vi "FaulhaberV3-Ascii_V1.vi"() -> (1 "searchnames":string[](array[string]), 2 "ID":u32[](array[numeric]), 3 "Faulhaber Objects":T3(array[cluster]))   [LabVIEW 2011] (continued)
ype=\"7\" dataType=\"0005\" lowLimit=\"0\" highLimit=\"128\" accessType=\"rw\" defaultValue=\"0\" PDOmapping=\"RPDO\" objFlags=\"00020000\" />\n\t\t\t\t\t\t<CANopenSubObject subIndex=\"02\" name=\"Current feedforward delay\" objectType=\"7\" dataType=\"0006\" lowLimit=\"0\" highLimit=\"65535\" accessType=\"rw\" defaultValue=\"0\" PDOmapping=\"no\" objFlags=\"00020000\" />\n\t\t\t\t\t</CANopenObject>\n\t\t\t\t\t<CANopenObject index=\"234A\" name=\"Velocity feedforward parameters\" objectType=\"9\" subNumber=\"3\">\n\t\t\t\t\t\t<CANopenSubObject subIndex=\"00\" name=\"Number of entries\" objectType=\"7\" dataType=\"0005\" accessType=\"ro\" defaultValue=\"2\" PDOmapping=\"no\" />\n\t\t\t\t\t\t<CANopenSubObject subIndex=\"01\" name=\"Velocity feedforward factor\" objectType=\"7\" dataType=\"0005\" lowLimit=\"0\" highLimit=\"128\" accessType=\"rw\" defaultValue=\"0\" PDOmapping=\"RPDO\" objFlags=\"00020000\" />\n\t\t\t\t\t\t<CANopenSubObject subIndex=\"02\" name=\"Velocity feedforward delay\" objectType=\"7\" dataType=\"0006\" lowLimit=\"0\" highLimit=\"65535\" accessType=\"rw\" defaultValue=\"0\" PDOmapping=\"no\" objFlags=\"00020000\" />\n\t\t\t\t\t</CANopenObject>\n\t\t\t\t\t<CANopenObject index=\"234B\" name=\"Current filter parameters\" objectType=\"9\" subNumber=\"3\">\n\t\t\t\t\t\t<CANopenSubObject subIndex=\"00\" name=\"Number of entries\" objectType=\"7\" dataType=\"0005\" accessType=\"ro\" defaultValue=\"2\" PDOmapping=\"no\" />\n\t\t\t\t\t\t<CANopenSubObject subIndex=\"01\" name=\"Display current filter TF\" objectType=\"7\" dataType=\"0006\" lowLimit=\"0\" highLimit=\"65535\" accessType=\"rw\" PDOmapping=\"RPDO\" objFlags=\"00020000\" />\n\t\t\t\t\t\t<CANopenSubObject subIndex=\"02\" name=\"Display torque filter TF\" objectType=\"7\" dataType=\"0006\" lowLimit=\"0\" highLimit=\"65535\" accessType=\"rw\" PDOmapping=\"RPDO\" objFlags=\"00020000\" />\n\t\t\t\t\t</CANopenObject>\n\t\t\t\t\t<CANopenObject index=\"234C\" name=\"Current compensation parameters\" objectType=\"9\" subNumber=\"4\">\n\t\t\t\t\t\t<CANopenSubObject subIndex=\"00\" name=\"Number of entries\" objectType=\"7\" dataType=\"0005\" accessType=\"ro\" defaultValue=\"3\" PDOmapping=\"no\" />\n\t\t\t\t\t\t<CANopenSubObject subIndex=\"01\" name=\"Gravity compensation\" objectType=\"7\" dataType=\"0003\" lowLimit=\"-32768\" highLimit=\"32767\" accessType=\"rw\" defaultValue=\"0\" PDOmapping=\"RPDO\" objFlags=\"00020000\" />\n\t\t\t\t\t\t<CANopenSubObject subIndex=\"02\" name=\"Positive friction compensation\" objectType=\"7\" dataType=\"0006\" lowLimit=\"0\" highLimit=\"6000\" accessType=\"rw\" defaultValue=\"0\" PDOmapping=\"RPDO\" objFlags=\"00020000\" />\n\t\t\t\t\t\t<CANopenSubObject subIndex=\"03\" name=\"Negative friction compensation\" objectType=\"7\" dataType=\"0006\" lowLimit=\"0\" highLimit=\"6000\" accessType=\"rw\" defaultValue=\"0\" PDOmapping=\"RPDO\" objFlags=\"00020000\" />\n\t\t\t\t\t</CANopenObject>\n\t\t\t\t\t<CANopenObject index=\"2350\" name=\"Positive torque limit homing\" objectType=\"7\" dataType=\"0006\" lowLimit=\"0\" highLimit=\"6000\" accessType=\"rw\" defaultValue=\"1000\" PDOmapping=\"RPDO\" objFlags=\"00020000\" />\n\t\t\t\t\t<CANopenObject index=\"2351\" name=\"Negative torque limit homing\" objectType=\"7\" dataType=\"0006\" lowLimit=\"0\" highLimit=\"6000\" accessType=\"rw\" defaultValue=\"1000\" PDOmapping=\"RPDO\" objFlags=\"00020000\" />\n\t\t\t\t\t<CANopenObject index=\"2360\" name=\"Actual values\" objectType=\"9\" subNumber=\"11\">\n\t\t\t\t\t\t<CANopenSubObject subIndex=\"00\" name=\"Number of entries\" objectType=\"7\" dataType=\"0005\" accessType=\"ro\" defaultValue=\"10\" PDOmapping=\"no\" />\n\t\t\t\t\t\t<CANopenSubObject subIndex=\"01\" name=\"Motor current Id actual value\" objectType=\"7\" dataType=\"0003\" accessType=\"ro\" PDOmapping=\"TPDO\" />\n\t\t\t\t\t\t<CANopenSubObject subIndex=\"02\" name=\"Motor current Iq actual value\" objectType=\"7\" dataType=\"0003\" accessType=\"ro\" PDOmapping=\"TPDO\" />\n\t\t\t\t\t\t<CANopenSubObject subIndex=\"03\" name=\"Motor currrent IBlock actual value\" objectType=\"7\" dataType=\"0003\" accessType=\"ro\" PDOmapping=\"TPDO\" />\n\t\t\t\t\t\t<CANopenSubObject subIndex=\"04\" name=\"Motor current IDC actual value\" objectType=\"7\" dataType=\"0003\" accessType=\"ro\" PDOmapping=\"TPDO\" />\n\t\t\t\t\t\t<CANopenSubObject subIndex=\"05\" name=\"Velocity actual internal value\" objectType=\"7\" dataType=\"0003\" accessType=\"ro\" PDOmapping=\"TPDO\" />\n\t\t\t\t\t\t<CANopenSubObject subIndex=\"06\" name=\"Position actual internal value\" objectType=\"7\" dataType=\"0004\" accessType=\"ro\" PDOmapping=\"TPDO\" />\n\t\t\t\t\t\t<CANopenSubObject subIndex=\"07\" name=\"Actual commutation segment\" objectType=\"7\" dataType=\"0005\" accessType=\"ro\" PDOmapping=\"TPDO\" />\n\t\t\t\t\t\t<CANopenSubObject subIndex=\"08\" name=\"Actual commutation angle\" objectType=\"7\" dataType=\"0003\" accessType=\"ro\" PDOmapping=\"TPDO\" />\n\t\t\t\t\t\t<CANopenSubObject subIndex=\"09\" name=\"Reserved 9\" objectType=\"7\" dataType=\"0004\" accessType=\"ro\" PDOmapping=\"TPDO\" objFlags=\"00020003\" />\n\t\t\t\t\t\t<CANopenSubObject subIndex=\"0A\" name=\"Reserved 10\" objectType=\"7\" dataType=\"0004\" lowLimit=\"-2147483648\" highLimit=\"2147483647\" accessType=\"wo\" PDOmapping=\"no\" objFlags=\"00020003\" />\n\t\t\t\t\t</CANopenObject>\n\t\t\t\t\t<CANopenObject index=\"2370\" name=\"Trace configuration\" objectType=\"9\" subNumber=\"16\">\n\t\t\t\t\t\t<CANopenSubObject subIndex=\"00\" name=\"Number of entries\" objectType=\"7\" dataType=\"0005\" accessType=\"ro\" defaultValue=\"15\" PDOmapping=\"no\" />\n\t\t\t\t\t\t<CANopenSubObject subIndex=\"01\" name=\"Trigger value\" objectType=\"7\" dataType=\"0007\" lowLimit=\"0\" highLimit=\"4294967295\" accessType=\"rw\" defaultValue=\"0x00\" PDOmapping=\"no\" objFlags=\"00020000\" />\n\t\t\t\t\t\t<CANopenSubObject subIndex=\"02\" name=\"Trigger threshold\" objectType=\"7\" dataType=\"0004\" lowLimit=\"-2147483648\" highLimit=\"2147483647\" accessType=\"rw\" defaultValue=\"0\" PDOmapping=\"no\" objFlags=\"00020000\" />\n\t\t\t\t\t\t<CANopenSubObject subIndex=\"03\" name=\"Trigger offset\" objectType=\"7\" dataType=\"0003\" lowLimit=\"-32768\" highLimit=\"32767\" accessType=\"rw\" defaultValue=\"0\" PDOmapping=\"no\" objFlags=\"00020000\" />\n\t\t\t\t\t\t<CANopenSubObject subIndex=\"04\" name=\"Trigger mode\" objectType=\"7\" dataType=\"0006\" lowLimit=\"0\" highLimit=\"65535\" accessType=\"rw\" defaultValue=\"0\" PDOmapping=\"no\" objFlags=\"00020000\" />\n\t\t\t\t\t\t<CANopenSubObject subIndex=\"05\" name=\"Buffer length\" objectType=\"7\" dataType=\"0006\" lowLimit=\"1\" highLimit=\"2048\" accessType=\"rw\" defaultValue=\"2048\" PDOmapping=\"no\" objFlags=\"00020000\" />\n\t\t\t\t\t\t<CANopenSubObject subIndex=\"06\" name=\"Sample time\" objectType=\"7\" dataType=\"0005\" lowLimit=\"1\" highLimit=\"255\" accessType=\"rw\" defaultValue=\"1\" PDOmapping=\"no\" objFlags=\"00020000\" />\n\t\t\t\t\t\t<CANopenSubObject subIndex=\"07\" name=\"Trace source of channel 1\" objectType=\"7\" dataType=\"0007\" lowLimit=\"0\" highLimit=\"4294967295\" accessType=\"rw\" defaultValue=\"0x00\" PDOmapping=\"no\" objFlags=\"00020000\" />\n\t\t\t\t\t\t<CANopenSubObject subIndex=\"08\" name=\"Trace source of channel 2\" objectType=\"7\" dataType=\"0007\" lowLimit=\"0\" highLimit=\"4294967295\" accessType=\"rw\" defaultValue=\"0x00\" PDOmapping=\"no\" objFlags=\"00020000\" />\n\t\t\t\t\t\t<CANopenSubObject subIndex=\"09\" name=\"Trace source of channel 3\" objectType=\"7\" dataType=\"0007\" lowLimit=\"0\" highLimit=\"4294967295\" accessType=\"rw\" defaultValue=\"0x00\" PDOmapping=\"no\" objFlags=\"00020000\" />\n\t\t\t\t\t\t<CANopenSubObject subIndex=\"0A\" name=\"Trace source of channel 4\" objectType=\"7\" dataType=\"0007\" lowLimit=\"0\" highLimit=\"4294967295\" accessType=\"rw\" defaultValue=\"0x00\" PDOmapping=\"no\" objFlags=\"00020000\" />\n\t\t\t\t\t\t<CANopenSubObject subIndex=\"0B\" name=\"Monitor source of channel 1\" objectType=\"7\" dataType=\"0007\" lowLimit=\"0\" highLimit=\"4294967295\" accessType=\"rw\" defaultValue=\"0x00\" PDOmapping=\"no\" objFlags=\"00020000\" />\n\t\t\t\t\t\t<CANopenSubObject subIndex=\"0C\" name=\"Monitor source of channel 2\" objectType=\"7\" dataType=\"0007\" lowLimit=\"0\" highLimit=\"4294967295\" accessType=\"rw\" defaultValue=\"0x00\" PDOmapping=\"no\" objFlags=\"00020000\" />\n\t\t\t\t\t\t<CANopenSubObject subIndex=\"0D\" name=\"Monitor source of channel 3\" objectType=\"7\" dataType=\"0007\" lowLimit=\"0\" highLimit=\"4294967295\" accessType=\"rw\" defaultValue=\"0x00\" PDOmapping=\"no\" objFlags=\"00020000\" />\n\t\t\t\t\t\t<CANopenSubObject subIndex=\"0E\" name=\"Monitor source of channel 4\" objectType=\"7\" dataType=\"0007\" lowLimit=\"0\" highLimit=\"4294967295\" accessType=\"rw\" defaultValue=\"0x00\" PDOmapping=\"no\" objFlags=\"00020000\" />\n\t\t\t\t\t\t<CANopenSubObject subIndex=\"0F\" name=\"Extended recorder mode\" objectType=\"7\" dataType=\"0006\" lowLimit=\"0\" highLimit=\"65535\" accessType=\"wo\" defaultValue=\"0x00\" PDOmapping=\"no\" objFlags=\"00020000\" />\n\t\t\t\t\t</CANopenObject>\n\t\t\t\t\t<CANopenObject index=\"2371\" name=\"Trace buffer\" objectType=\"9\" subNumber=\"6\">\n\t\t\t\t\t\t<CANopenSubObject subIndex=\"00\" name=\"Number of entries\" objectType=\"7\" dataType=\"0005\" accessType=\"ro\" defaultValue=\"5\" PDOmapping=\"no\" />\n\t\t\t\t\t\t<CANopenSubObject subIndex=\"01\" name=\"Trace state\" objectType=\"7\" dataType=\"0006\" accessType=\"ro\" PDOmapping=\"no\" />\n\t\t\t\t\t\t<CANopenSubObject subIndex=\"02\" name=\"Trace value of channel 1\" objectType=\"2\" dataType=\"0009\" accessType=\"ro\" PDOmapping=\"no\" objFlags=\"0002\" />\n\t\t\t\t\t\t<CANopenSubObject subIndex=\"03\" name=\"Trace value of channel 2\" objectType=\"2\" dataType=\"0009\" accessType=\"ro\" PDOmapping=\"no\" objFlags=\"0002\" />\n\t\t\t\t\t\t<CANopenSubObject subIndex=\"04\" name=\"Trace value of channel 3\" objectType=\"2\" dataType=\"0009\" accessType=\"ro\" PDOmapping=\"no\" objFlags=\"0002\" />\n\t\t\t\t\t\t<CANopenSubObject subIndex=\"05\" name=\"Trace value of channel 4\" objectType=\"2\" dataType=\"0009\" accessType=\"ro\" PDOmapping=\"no\" objFlags=\"0002\" />\n\t\t\t\t\t</CANopenObject>\n\t\t\t\t\t<CANopenObject index=\"2372\" name=\"Logic trigger configuration\" objectType=\"9\" subNumber=\"3\">\n\t\t\t\t\t\t<CANopenSubObject subIndex=\"00\" name=\"Number of entries\" objectType=\"7\" dataType=\"0005\" accessType=\"ro\" defaultValue=\"2\" PDOmapping=\"no\" />\n\t\t\t\t\t\t<CANopenSubObject subIndex=\"01\" name=\"Logic trigger AND mask\" objectType=\"7\" dataType=\"0007\" lowLimit=\"0\" highLimit=\"4294967295\" accessType=\"rw\" defaultValue=\"0x00\" PDOmapping=\"no\" objFlags=\"00020000\" />\n\t\t\t\t\t\t<CANopenSubObject subIndex=\"02\" name=\"Logic trigger OR mask\" objectType=\"7\" dataType=\"0007\" lowLimit=\"0\" highLimit=\"4294967295\" accessType=\"rw\" defaultValue=\"0x00\" PDOmapping=\"no\" objFlags=\"00020000\" />\n\t\t\t\t\t</CANopenObject>\n\t\t\t\t\t<CANopenObject index=\"2373\" name=\"Event trigger configuration\" objectType=\"9\" subNumber=\"2\">\n\t\t\t\t\t\t<CANopenSubObject subIndex=\"00\" name=\"Number of entries\" objectType=\"7\" dataType=\"0005\" accessType=\"ro\" defaultValue=\"1\" PDOmapping=\"no\" />\n\t\t\t\t\t\t<CANopenSubObject subIndex=\"01\" name=\"Event trigger event selection\" objectType=\"7\" dataType=\"0006\" PDOmapping=\"no\" objFlags=\"00020000\" uniqueIDRef=\"UID_PARAM_237301\" />\n\t\t\t\t\t</CANopenObject>\n\t\t\t\t\t<CANopenObject index=\"2374\" name=\"Event flag configuration\" objectType=\"9\" subNumber=\"3\">\n\t\t\t\t\t\t<CANopenSubObject subIndex=\"00\" name=\"Number of entries\" objectType=\"7\" dataType=\"0005\" accessType=\"ro\" defaultValue=\"2\" PDOmapping=\"no\" />\n\t\t\t\t\t\t<CANopenSubObject subIndex=\"01\" name=\"Event flag set mask\" objectType=\"7\" dataType=\"0006\" lowLimit=\"0\" highLimit=\"65535\" accessType=\"rw\" defaultValue=\"0x0\" PDOmapping=\"no\" objFlags=\"00020000\" />\n\t\t\t\t\t\t<CANopenSubObject subIndex=\"02\" name=\"Event flag reset mask\" objectType=\"7\" dataType=\"0006\" lowLimit=\"0\" highLimit=\"65535\" accessType=\"rw\" defaultValue=\"0x0\" PDOmapping=\"no\" objFlags=\"00020000\" />\n\t\t\t\t\t</CANopenObject>\n\t\t\t\t\t<CANopenObject index=\"2378\" name=\"Trace channel configuration\" objectType=\"9\" subNumber=\"18\">\n\t\t\t\t\t\t<CANopenSubObject subIndex=\"00\" name=\"Number of entries\" objectType=\"7\" dataType=\"0005\" accessType=\"ro\" defaultValue=\"23\" PDOmapping=\"no\" />\n\t\t\t\t\t\t<CANopenSubObject subIndex=\"01\" name=\"Channel 1 filter time\" objectType=\"7\" dataType=\"0006\" lowLimit=\"0\" highLimit=\"65535\" accessType=\"rw\" defaultValue=\"0\" PDOmapping=\"RPDO\" objFlags=\"00020000\" />\n\t\t\t\t\t\t<CANopenSubObject subIndex=\"02\" name=\"Channel 1 sample time\" objectType=\"7\" dataType=\"0006\" lowLimit=\"0\" highLimit=\"65535\" accessType=\"rw\" defaultValue=\"1\" PDOmapping=\"RPDO\" objFlags=\"00020000\" />\n\t\t\t\t\t\t<CANopenSubObject subIndex=\"03\" name=\"Channel 1 number of samples\" objectType=\"7\" dataType=\"0006\" lowLimit=\"0\" highLimit=\"65535\" accessType=\"rw\" defaultValue=\"512\" PDOmapping=\"RPDO\" objFlags=\"00020000\" />\n\t\t\t\t\t\t<CANopenSubObject subIndex=\"04\" name=\"Channel 1 monitoring values\" objectType=\"7\" dataType=\"0006\" lowLimit=\"0\" highLimit=\"0x003F\" accessType=\"rw\" defaultValue=\"0\" PDOmapping=\"RPDO\" objFlags=\"00020000\" />\n\t\t\t\t\t\t<CANopenSubObject subIndex=\"05\" name=\"Channel 1 start event selection\" objectType=\"7\" dataType=\"0005\" PDOmapping=\"RPDO\" objFlags=\"00020000\" uniqueIDRef=\"UID_PARAM_237805\" />\n\t\t\t\t\t\t<CANopenSubObject subIndex=\"06\" name=\"Channel 1 update event selection\" objectType=\"7\" dataType=\"0005\" PDOmapping=\"RPDO\" objFlags=\"00020000\" uniqueIDRef=\"UID_PARAM_237806\" />\n\t\t\t\t\t\t<CANopenSubObject subIndex=\"07\" name=\"Channel 1 number of eval-cycles\" objectType=\"7\" dataType=\"0007\" lowLimit=\"0\" highLimit=\"4294967295\" accessType=\"rw\" defaultValue=\"0\" PDOmapping=\"TPDO\" objFlags=\"00020000\" />\n\t\t\t\t\t\t<CANopenSubObject subIndex=\"0E\" name=\"Channel 1 number of turnovers\" objectType=\"7\" dataType=\"0007\" accessType=\"ro\" PDOmapping=\"TPDO\" objFlags=\"00020000\" />\n\t\t\t\t\t\t<CANopenSubObject subIndex=\"0F\" name=\"Channel 1 done\" objectType=\"7\" dataType=\"0005\" accessType=\"ro\" PDOmapping=\"TPDO\" />\n\t\t\t\t\t\t<CANopenSubObject subIndex=\"10\" name=\"Channel 1 abs min value\" objectType=\"7\" dataType=\"0004\" accessType=\"ro\" defaultValue=\"2147483647\" PDOmapping=\"TPDO\" />\n\t\t\t\t\t\t<CANopenSubObject subIndex=\"11\" name=\"Channel 1 abs max value\" objectType=\"7\" dataType=\"0004\" accessType=\"ro\" defaultValue=\"-2147483648\" PDOmapping=\"TPDO\" />\n\t\t\t\t\t\t<CANopenSubObject subIndex=\"12\" name=\"Channel 1 minimum\" objectType=\"7\" dataType=\"0004\" accessType=\"ro\" PDOmapping=\"TPDO\" />\n\t\t\t\t\t\t<CANopenSubObject subIndex=\"13\" name=\"Channel 1 maximum\" objectType=\"7\" dataType=\"0004\" accessType=\"ro\" PDOmapping=\"TPDO\" />\n\t\t\t\t\t\t<CANopenSubObject subIndex=\"14\" name=\"Channel 1 mean value\" objectType=\"7\" dataType=\"0004\" accessType=\"ro\" PDOmapping=\"TPDO\" />\n\t\t\t\t\t\t<CANopenSubObject subIndex=\"15\" name=\"Channel 1 rms value\" objectType=\"7\" dataType=\"0004\" accessType=\"ro\" PDOmapping=\"TPDO\" />\n\t\t\t\t\t\t<CANopenSubObject subIndex=\"16\" name=\"Channel 1 period time\" objectType=\"7\" dataType=\"0007\" accessType=\"ro\" PDOmapping=\"TPDO\" />\n\t\t\t\t\t\t<CANopenSubObject subIndex=\"17\" name=\"Channel 1 sigma\" objectType=\"7\" dataType=\"0004\" accessType=\"ro\" PDOmapping=\"TPDO\" />\n\t\t\t\t\t</CANopenObject>\n\t\t\t\t\t<CANopenObject index=\"2379\" name=\"Trace channel configuration\" objectType=\"9\" subNumber=\"18\">\n\t\t\t\t\t\t<CANopenSubObject subIndex=\"00\" name=\"Number of entries\" objectType=\"7\" dataType=\"0005\" accessType=\"ro\" defaultValue=\"23\" PDOmapping=\"no\" />\n\t\t\t\t\t\t<CANopenSubObject subIndex=\"01\" name=\"Channel 2 filter time\" objectType=\"7\" dataType=\"0006\" lowLimit=\"0\" highLimit=\"65535\" accessType=\"rw\" defaultValue=\"0\" PDOmapping=\"RPDO\" objFlags=\"00020000\" />\n\t\t\t\t\t\t<CANopenSubObject subIndex=\"02\" name=\"Channel 2 sample time\" objectType=\"7\" dataType=\"0006\" lowLimit=\"0\" highLimit=\"65535\" accessType=\"rw\" defaultValue=\"1\" PDOmapping=\"RPDO\" objFlags=\"00020000\" />\n\t\t\t\t\t\t<CANopenSubObject subIndex=\"03\" name=\"Channel 2 number of samples\" objectType=\"7\" dataType=\"0006\" lowLimit=\"0\" highLimit=\"65535\" accessType=\"rw\" defaultValue=\"512\" PDOmapping=\"RPDO\" objFlags=\"00020000\" />\n\t\t\t\t\t\t<CANopenSubObject subIndex=\"04\" name=\"Channel 2 monitoring values\" objectType=\"7\" dataType=\"0006\" lowLimit=\"0\" highLimit=\"0x003F\" accessType=\"rw\" defaultValue=\"0\" PDOmapping=\"RPDO\" objFlags=\"00020000\" />\n\t\t\t\t\t\t<CANopenSubObject subIndex=\"05\" name=\"Channel 2 startevent selection\" objectType=\"7\" dataType=\"0005\" PDOmapping=\"RPDO\" objFlags=\"00020000\" uniqueIDRef=\"UID_PARAM_237905\" />\n\t\t\t\t\t\t<CANopenSubObject subIndex=\"06\" name=\"Channel 2 update event selection\" objectType=\"7\" dataType=\"0005\" PDOmapping=\"RPDO\" objFlags=\"00020000\" uniqueIDRef=\"UID_PARAM_237906\" />\n\t\t\t\t\t\t<CANopenSubObject subIndex=\"07\" name=\"Channel 2 number of eval-cycles\" objectType=\"7\" dataType=\"0007\" lowLimit=\"0\" highLimit=\"4294967295\" accessType=\"rw\" defaultValue=\"0\" PDOmapping=\"TPDO\" objFlags=\"00020000\" />\n\t\t\t\t\t\t<CANopenSubObject subIndex=\"0E\" name=\"Channel 2 number of turn-overs\" objectType=\"7\" dataType=\"0007\" accessType=\"ro\" PDOmapping=\"TPDO\" objFlags=\"00020000\" />\n\t\t\t\t\t\t<CANopenSubObject subIndex=\"0F\" name=\"Channel 2 done\" objectType=\"7\" dataType=\"0005\" accessType=\"ro\" PDOmapping=\"TPDO\" />\n\t\t\t\t\t\t<CANopenSubObject subIndex=\"10\" name=\"Channel 2 abs min value\" objectType=\"7\" dataType=\"0004\" accessType=\"ro\" defaultValue=\"2147483647\" PDOmapping=\"TPDO\" />\n\t\t\t\t\t\t<CANopenSubObject subIndex=\"11\" name=\"Channel 2 abs max value\" objectType=\"7\" dataType=\"0004\" accessType=\"ro\" defaultValue=\"-2147483648\" PDOmapping=\"TPDO\" />\n\t\t\t\t\t\t<CANopenSubObject subIndex=\"12\" name=\"Channel 2 minimum\" objectType=\"7\" dataType=\"0004\" accessType=\"ro\" PDOmapping=\"TPDO\" />\n\t\t\t\t\t\t<CANopenSubObject subIndex=\"13\" name=\"Channel 2 maximum\" objectType=\"7\" dataType=\"0004\" accessType=\"ro\" PDOmapping=\"TPDO\" />\n\t\t\t\t\t\t<CANopenSubObject subIndex=\"14\" name=\"Channel 2 mean value\" objectType=\"7\" dataType=\"0004\" accessType=\"ro\" PDOmapping=\"TPDO\" />\n\t\t\t\t\t\t<CANopenSubObject subIndex=\"15\" name=\"Channel 2 rms value\" objectType=\"7\" dataType=\"0004\" accessType=\"ro\" PDOmapping=\"TPDO\" />\n\t\t\t\t\t\t<CANopenSubObject subIndex=\"16\" name=\"Channel 2 period time\" objectType=\"7\" dataType=\"0007\" accessType=\"ro\" PDOmapping=\"TPDO\" />\n\t\t\t\t\t\t<CANopenSubObject subIndex=\"17\" name=\"Channel 2 sigma\" objectType=\"7\" dataType=\"0004\" accessType=\"ro\" PDOmapping=\"TPDO\" />\n\t\t\t\t\t</CANopenObject>\n\t\t\t\t\t<CANopenObject index=\"237A\" name=\"Trace channel configuration\" objectType=\"9\" subNumber=\"18\">\n\t\t\t\t\t\t<CANopenSubObject subIndex=\"00\" name=\"Number of entries\" objectType=\"7\" dataType=\"0005\" accessType=\"ro\" defaultValue=\"23\" PDOmapping=\"no\" />\n\t\t\t\t\t\t<CANopenSubObject subIndex=\"01\" name=\"Channel 3 filter time\" objectType=\"7\" dataType=\"0006\" lowLimit=\"0\" highLimit=\"65535\" accessType=\"rw\" defaultValue=\"0\" PDOmapping=\"RPDO\" objFlags=\"00020000\" />\n\t\t\t\t\t\t<CANopenSubObject subIndex=\"02\" name=\"Channel 3 sample time\" objectType=\"7\" dataType=\"0006\" lowLimit=\"0\" highLimit=\"65535\" accessType=\"rw\" defaultValue=\"1\" PDOmapping=\"RPDO\" objFlags=\"00020000\" />\n\t\t\t\t\t\t<CANopenSubObject subIndex=\"03\" name=\"Channel 3 number of samples\" objectType=\"7\" dataType=\"0006\" lowLimit=\"0\" highLimit=\"65535\" accessType=\"rw\" defaultValue=\"512\" PDOmapping=\"RPDO\" objFlags=\"00020000\" />\n\t\t\t\t\t\t<CANopenSubObject subIndex=\"04\" name=\"Channel 3 monitoring values\" objectType=\"7\" dataType=\"0006\" lowLimit=\"0\" highLimit=\"0x003F\" accessType=\"rw\" defaultValue=\"0\" PDOmapping=\"RPDO\" objFlags=\"00020000\" />\n\t\t\t\t\t\t<CANopenSubObject subIndex=\"05\" name=\"Channel 3 start event selection\" objectType=\"7\" dataType=\"0005\" PDOmapping=\"RPDO\" objFlags=\"00020000\" uniqueIDRef=\"UID_PARAM_237A05\" />\n\t\t\t\t\t\t<CANopenSubObject subIndex=\"06\" name=\"Channel 3 update event selection\" objectType=\"7\" dataType=\"0005\" PDOmapping=\"RPDO\" objFlags=\"00020000\" uniqueIDRef=\"UID_PARAM_237A06\" />\n\t\t\t\t\t\t<CANopenSubObject subIndex=\"07\" name=\"Channel 3 number of eval-cycles\" objectType=\"7\" dataType=\"0007\" lowLimit=\"0\" highLimit=\"4294967295\" accessType=\"rw\" defaultValue=\"0\" PDOmapping=\"TPDO\" objFlags=\"00020000\" />\n\t\t\t\t\t\t<CANopenSubObject subIndex=\"0E\" name=\"Channel 3 number of turn-overs\" objectType=\"7\" dataType=\"0007\" accessType=\"ro\" PDOmapping=\"TPDO\" objFlags=\"00020000\" />\n\t\t\t\t\t\t<CANopenSubObject subIndex=\"0F\" name=\"Channel 3 done\" objectType=\"7\" dataType=\"0005\" accessType=\"ro\" PDOmapping=\"TPDO\" />\n\t\t\t\t\t\t<CANopenSubObject subIndex=\"10\" name=\"Channel 3 abs min value\" objectType=\"7\" dataType=\"0004\" accessType=\"ro\" defaultValue=\"2147483647\" PDOmapping=\"TPDO\" />\n\t\t\t\t\t\t<CANopenSubObject subIndex=\"11\" name=\"Channel 3 abs max value\" objectType=\"7\" dataType=\"0004\" accessType=\"ro\" defaultValue=\"-2147483648\" PDOmapping=\"TPDO\" />\n\t\t\t\t\t\t<CANopenSubObject subIndex=\"12\" name=\"Channel 3 minimum\" objectType=\"7\" dataType=\"0004\" accessType=\"ro\" PDOmapping=\"TPDO\" />\n\t\t\t\t\t\t<CANopenSubObject subIndex=\"13\" name=\"Channel 3 maximum\" objectType=\"7\" dataType=\"0004\" accessType=\"ro\" PDOmapping=\"TPDO\" />\n\t\t\t\t\t\t<CANopenSubObject subIndex=\"14\" name=\"Channel 3 mean value\" objectType=\"7\" dataType=\"0004\" accessType=\"ro\" PDOmapping=\"TPDO\" />\n\t\t\t\t\t\t<CANopenSubObject subIndex=\"15\" name=\"Channel 3 rms value\" objectType=\"7\" dataType=\"0004\" accessType=\"ro\" PDOmapping=\"TPDO\" />\n\t\t\t\t\t\t<CANopenSubObject subIndex=\"16\" name=\"Channel 3 period time\" objectType=\"7\" dataType=\"0007\" accessType=\"ro\" PDOmapping=\"TPDO\" />\n\t\t\t\t\t\t<CANopenSubObject subIndex=\"17\" name=\"Channel 3 sigma\" objectType=\"7\" dataType=\"0004\" accessType=\"ro\" PDOmapping=\"TPDO\" />\n\t\t\t\t\t</CANopenObject>\n\t\t\t\t\t<CANopenObject index=\"237B\" name=\"Trace channel configuration\" objectType=\"9\" subNumber=\"18\">\n\t\t\t\t\t\t<CANopenSubObject subIndex=\"00\" name=\"Number of entries\" objectType=\"7\" dataType=\"0005\" accessType=\"ro\" defaultValue=\"23\" PDOmapping=\"no\" />\n\t\t\t\t\t\t<CANopenSubObject subIndex=\"01\" name=\"Channel 4 filter time\" objectType=\"7\" dataType=\"0006\" lowLimit=\"0\" highLimit=\"65535\" accessType=\"rw\" defaultValue=\"0\" PDOmapping=\"RPDO\" objFlags=\"00020000\" />\n\t\t\t\t\t\t<CANopenSubObject subIndex=\"02\" name=\"Channel 4 sample time\" objectType=\"7\" dataType=\"0006\" lowLimit=\"0\" highLimit=\"65535\" accessType=\"rw\" defaultValue=\"1\" PDOmapping=\"RPDO\" objFlags=\"00020000\" />\n\t\t\t\t\t\t<CANopenSubObject subIndex=\"03\" name=\"Channel 4 number of samples\" objectType=\"7\" dataType=\"0006\" lowLimit=\"0\" highLimit=\"65535\" accessType=\"rw\" defaultValue=\"512\" PDOmapping=\"RPDO\" objFlags=\"00020000\" />\n\t\t\t\t\t\t<CANopenSubObject subIndex=\"04\" name=\"Channel 4 monitoring values\" objectType=\"7\" dataType=\"0006\" lowLimit=\"0\" highLimit=\"0x003F\" accessType=\"rw\" defaultValue=\"0\" PDOmapping=\"RPDO\" objFlags=\"00020000\" />\n\t\t\t\t\t\t<CANopenSubObject subIndex=\"05\" name=\"Channel 4 start event selection\" objectType=\"7\" dataType=\"0005\" PDOmapping=\"RPDO\" objFlags=\"00020000\" uniqueIDRef=\"UID_PARAM_237B05\" />\n\t\t\t\t\t\t<CANopenSubObject subIndex=\"06\" name=\"Channel 4 update event selection\" objectType=\"7\" dataType=\"0005\" PDOmapping=\"RPDO\" objFlags=\"00020000\" uniqueIDRef=\"UID_PARAM_237B06\" />\n\t\t\t\t\t\t<CANopenSubObject subIndex=\"07\" name=\"Channel 4 number of eval-cycles\" objectType=\"7\" dataType=\"0007\" lowLimit=\"0\" highLimit=\"4294967295\" accessType=\"rw\" defaultValue=\"0\" PDOmapping=\"TPDO\" objFlags=\"00020000\" />\n\t\t\t\t\t\t<CANopenSubObject subIndex=\"0E\" name=\"Channel 4 number of turn-overs\" objectType=\"7\" dataType=\"0007\" accessType=\"ro\" PDOmapping=\"TPDO\" objFlags=\"00020000\" />\n\t\t\t\t\t\t<CANopenSubObject subIndex=\"0F\" name=\"Channel 4 done\" objectType=\"7\" dataType=\"0005\" accessType=\"ro\" PDOmapping=\"TPDO\" />\n\t\t\t\t\t\t<CANopenSubObject subIndex=\"10\" name=\"Channel 4 abs min value\" objectType=\"7\" dataType=\"0004\" accessType=\"ro\" defaultValue=\"2147483647\" PDOmapping=\"TPDO\" />\n\t\t\t\t\t\t<CANopenSubObject subIndex=\"11\" name=\"Channel 4 abs max value\" objectType=\"7\" dataType=\"0004\" accessType=\"ro\" defaultValue=\"-2147483648\" PDOmapping=\"TPDO\" />\n\t\t\t\t\t\t<CANopenSubObject subIndex=\"12\" name=\"Channel 4 minimum\" objectType=\"7\" dataType=\"0004\" accessType=\"ro\" PDOmapping=\"TPDO\" />\n\t\t\t\t\t\t<CANopenSubObject subIndex=\"13\" name=\"Channel 4 maximum\" objectType=\"7\" dataType=\"0004\" accessType=\"ro\" PDOmapping=\"TPDO\" />\n\t\t\t\t\t\t<CANopenSubObject subIndex=\"14\" name=\"Channel 4 mean value\" objectType=\"7\" dataType=\"0004\" accessType=\"ro\" PDOmapping=\"TPDO\" />\n\t\t\t\t\t\t<CANopenSubObject subIndex=\"15\" name=\"Channel 4 rms value\" objectType=\"7\" dataType=\"0004\" accessType=\"ro\" PDOmapping=\"TPDO\" />\n\t\t\t\t\t\t<CANopenSubObject subIndex=\"16\" name=\"Channel 4 period time\" objectType=\"7\" dataType=\"0007\" accessType=\"ro\" PDOmapping=\"TPDO\" />\n\t\t\t\t\t\t<CANopenSubObject subIndex=\"17\" name=\"Channel 4 sigma\" objectType=\"7\" dataType=\"0004\" accessType=\"ro\" PDOmapping=\"TPDO\" />\n\t\t\t\t\t</CANopenObject>\n\t\t\t\t\t<CANopenObject index=\"2380\" name=\"PRBS generator\" objectType=\"9\" subNumber=\"6\">\n\t\t\t\t\t\t<CANopenSubObject subIndex=\"00\" name=\"Number of entries\" objectType=\"7\" dataType=\"0005\" accessType=\"ro\" defaultValue=\"5\" PDOmapping=\"no\" objFlags=\"00020002\" />\n\t\t\t\t\t\t<CANopenSubObject subIndex=\"01\" name=\"Shift register init\" objectType=\"7\" dataType=\"0006\" lowLimit=\"0\" highLimit=\"65535\" accessType=\"rw\" PDOmapping=\"no\" objFlags=\"00020002\" />\n\t\t\t\t\t\t<CANopenSubObject subIndex=\"02\" name=\"Gain\" objectType=\"7\" dataType=\"0003\" lowLimit=\"-32768\" highLimit=\"32767\" accessType=\"rw\" PDOmapping=\"no\" objFlags=\"00020002\" />\n\t\t\t\t\t\t<CANopenSubObject subIndex=\"03\" name=\"Offset\" objectType=\"7\" dataType=\"0003\" lowLimit=\"-32768\" highLimit=\"32767\" accessType=\"rw\" PDOmapping=\"no\" objFlags=\"00020002\" />\n\t\t\t\t\t\t<CANopenSubObject subIndex=\"04\" name=\"Sample rate factor\" objectType=\"7\" dataType=\"0005\" lowLimit=\"0\" highLimit=\"255\" accessType=\"rw\" PDOmapping=\"no\" objFlags=\"00020002\" />\n\t\t\t\t\t\t<CANopenSubObject subIndex=\"05\" name=\"Enable\" objectType=\"7\" dataType=\"0005\" lowLimit=\"0\" highLimit=\"255\" accessType=\"rw\" PDOmapping=\"no\" objFlags=\"00020002\" />\n\t\t\t\t\t</CANopenObject>\n\t\t\t\t\t<CANopenObject index=\"2381\" name=\"Start up generator\" objectType=\"9\" subNumber=\"9\">\n\t\t\t\t\t\t<CANopenSubObject subIndex=\"00\" name=\"Number of entries\" objectType=\"7\" dataType=\"0005\" accessType=\"ro\" defaultValue=\"8\" PDOmapping=\"no\" objFlags=\"00020002\" />\n\t\t\t\t\t\t<CANopenSubObject subIndex=\"01\" name=\"Speed threshold\" objectType=\"7\" dataType=\"0006\" lowLimit=\"0\" highLimit=\"65535\" accessType=\"rw\" PDOmapping=\"no\" objFlags=\"00020002\" />\n\t\t\t\t\t\t<CANopenSubObject subIndex=\"02\" name=\"Timeout time\" objectType=\"7\" dataType=\"0007\" lowLimit=\"0\" highLimit=\"4294967295\" accessType=\"rw\" PDOmapping=\"no\" objFlags=\"00020002\" />\n\t\t\t\t\t\t<CANopenSubObject subIndex=\"03\" name=\"Target value\" objectType=\"7\" dataType=\"0006\" lowLimit=\"0\" highLimit=\"65535\" accessType=\"rw\" PDOmapping=\"no\" objFlags=\"00020002\" />\n\t\t\t\t\t\t<CANopenSubObject subIndex=\"04\" name=\"Reset\" objectType=\"7\" dataType=\"0005\" lowLimit=\"0\" highLimit=\"255\" accessType=\"rw\" PDOmapping=\"no\" objFlags=\"00020002\" />\n\t\t\t\t\t\t<CANopenSubObject subIndex=\"05\" name=\"Enable\" objectType=\"7\" dataType=\"0005\" lowLimit=\"0\" highLimit=\"255\" accessType=\"rw\" PDOmapping=\"no\" objFlags=\"00020002\" />\n\t\t\t\t\t\t<CANopenSubObject subIndex=\"06\" name=\"Ready\" objectType=\"7\" dataType=\"0007\" lowLimit=\"0\" highLimit=\"4294967295\" accessType=\"rw\" PDOmapping=\"no\" objFlags=\"00020002\" />\n\t\t\t\t\t\t<CANopenSubObject subIndex=\"07\" name=\"TimeThreshold\" objectType=\"7\" dataType=\"0007\" lowLimit=\"0\" highLimit=\"4294967295\" accessType=\"rw\" PDOmapping=\"no\" objFlags=\"00020002\" />\n\t\t\t\t\t\t<CANopenSubObject subIndex=\"08\" name=\"Iteration\" objectType=\"7\" dataType=\"0007\" lowLimit=\"0\" highLimit=\"4294967295\" accessType=\"rw\" PDOmapping=\"no\" objFlags=\"00020002\" />\n\t\t\t\t\t</CANopenObject>\n\t\t\t\t\t<CANopenObject index=\"2382\" name=\"Sinusoidal excitation\" objectType=\"9\" subNumber=\"4\">\n\t\t\t\t\t\t<CANopenSubObject subIndex=\"00\" name=\"Number of entries\" objectType=\"7\" dataType=\"0005\" accessType=\"ro\" defaultValue=\"3\" PDOmapping=\"no\" objFlags=\"00020002\" />\n\t\t\t\t\t\t<CANopenSubObject subIndex=\"01\" name=\"Amplitude\" objectType=\"7\" dataType=\"0006\" lowLimit=\"0\" highLimit=\"65535\" accessType=\"rw\" PDOmapping=\"no\" objFlags=\"00020002\" />\n\t\t\t\t\t\t<CANopenSubObject subIndex=\"02\" name=\"Frequency\" objectType=\"7\" dataType=\"0006\" lowLimit=\"0\" highLimit=\"65535\" accessType=\"rw\" PDOmapping=\"no\" objFlags=\"00020002\" />\n\t\t\t\t\t\t<CANopenSubObject subIndex=\"03\" name=\"Enable\" objectType=\"7\" dataType=\"0005\" lowLimit=\"0\" highLimit=\"255\" accessType=\"rw\" PDOmapping=\"no\" objFlags=\"00020002\" />\n\t\t\t\t\t</CANopenObject>\n\t\t\t\t\t<CANopenObject index=\"238F\" name=\"Select signal generator source\" objectType=\"9\" subNumber=\"2\">\n\t\t\t\t\t\t<CANopenSubObject subIndex=\"00\" name=\"Number of entries\" objectType=\"7\" dataType=\"0005\" accessType=\"ro\" defaultValue=\"1\" PDOmapping=\"no\" objFlags=\"00020002\" />\n\t\t\t\t\t\t<CANopenSubObject subIndex=\"01\" name=\"Selector\" objectType=\"7\" dataType=\"0005\" lowLimit=\"0\" highLimit=\"255\" accessType=\"rw\" defaultValue=\"0\" PDOmapping=\"no\" objFlags=\"00020002\" />\n\t\t\t\t\t</CANopenObject>\n\t\t\t\t\t<CANopenObject index=\"23F0\" name=\"23F0_00\" objectType=\"9\" subNumber=\"7\">\n\t\t\t\t\t\t<CANopenSubObject subIndex=\"00\" name=\"Number of entries\" objectType=\"7\" dataType=\"0005\" accessType=\"ro\" defaultValue=\"6\" PDOmapping=\"no\" objFlags=\"00020003\" />\n\t\t\t\t\t\t<CANopenSubObject subIndex=\"01\" name=\"23F0_01\" objectType=\"7\" dataType=\"0007\" accessType=\"ro\" PDOmapping=\"no\" objFlags=\"00020003\" />\n\t\t\t\t\t\t<CANopenSubObject subIndex=\"02\" name=\"23F0_02\" objectType=\"7\" dataType=\"0005\" accessType=\"ro\" PDOmapping=\"no\" objFlags=\"00020003\" />\n\t\t\t\t\t\t<CANopenSubObject subIndex=\"03\" name=\"23F0_03\" objectType=\"7\" dataType=\"0005\" accessType=\"ro\" PDOmapping=\"no\" objFlags=\"00020003\" />\n\t\t\t\t\t\t<CANopenSubObject subIndex=\"04\" name=\"23F0_04\" objectType=\"7\" dataType=\"0006\" accessType=\"ro\" PDOmapping=\"no\" objFlags=\"00020003\" />\n\t\t\t\t\t\t<CANopenSubObject subIndex=\"05\" name=\"23F0_05\" objectType=\"7\" dataType=\"0007\" accessType=\"ro\" PDOmapping=\"no\" objFlags=\"00020003\" />\n\t\t\t\t\t\t<CANopenSubObject subIndex=\"06\" name=\"23F0_06\" objectType=\"7\" dataType=\"0007\" accessType=\"ro\" PDOmapping=\"no\" objFlags=\"00020003\" />\n\t\t\t\t\t</CANopenObject>\n\t\t\t\t\t<CANopenObject index=\"23F1\" name=\"23F1_00\" objectType=\"9\" subNumber=\"3\">\n\t\t\t\t\t\t<CANopenSubObject subIndex=\"00\" name=\"Number of entries\" objectType=\"7\" dataType=\"0005\" accessType=\"ro\" defaultValue=\"2\" PDOmapping=\"no\" objFlags=\"00020003\" />\n\t\t\t\t\t\t<CANopenSubObject subIndex=\"01\" name=\"23F1_01\" objectType=\"7\" dataType=\"0004\" accessType=\"ro\" PDOmapping=\"no\" objFlags=\"00020003\" />\n\t\t\t\t\t\t<CANopenSubObject subIndex=\"02\" name=\"23F1_02\" objectType=\"7\" dataType=\"0004\" accessType=\"ro\" PDOmapping=\"no\" objFlags=\"00020003\" />\n\t\t\t\t\t</CANopenObject>\n\t\t\t\t\t<CANopenObject index=\"23F3\" name=\"23F2_00 \" objectType=\"9\" subNumber=\"6\">\n\t\t\t\t\t\t<CANopenSubObject subIndex=\"00\" name=\"Number of entries\" objectType=\"7\" dataType=\"0005\" accessType=\"ro\" defaultValue=\"5\" PDOmapping=\"no\" objFlags=\"0003\" />\n\t\t\t\t\t\t<CANopenSubObject subIndex=\"01\" name=\"Actual state\" objectType=\"7\" dataType=\"0002\" accessType=\"ro\" PDOmapping=\"no\" objFlags=\"0003\" />\n\t\t\t\t\t\t<CANopenSubObject subIndex=\"02\" name=\"Demand position\" objectType=\"7\" dataType=\"0004\" accessType=\"ro\" PDOmapping=\"no\" objFlags=\"0003\" />\n\t\t\t\t\t\t<CANopenSubObject subIndex=\"03\" name=\"Demand speed\" objectType=\"7\" dataType=\"0004\" accessType=\"ro\" PDOmapping=\"no\" objFlags=\"0003\" />\n\t\t\t\t\t\t<CANopenSubObject subIndex=\"04\" name=\"Demand acceleration\" objectType=\"7\" dataType=\"0003\" accessType=\"ro\" PDOmapping=\"no\" objFlags=\"0003\" />\n\t\t\t\t\t\t<CANopenSubObject subIndex=\"05\" name=\"Initial state\" objectType=\"7\" dataType=\"0002\" accessType=\"ro\" PDOmapping=\"no\" objFlags=\"0003\" />\n\t\t\t\t\t</CANopenObject>\n\t\t\t\t\t<CANopenObject index=\"2400\" name=\"Communication parameters\" objectType=\"9\" subNumber=\"8\">\n\t\t\t\t\t\t<CANopenSubObject subIndex=\"00\" name=\"Number of entries\" objectType=\"7\" dataType=\"0005\" accessType=\"ro\" defaultValue=\"7\" PDOmapping=\"no\" />\n\t\t\t\t\t\t<CANopenSubObject subIndex=\"01\" name=\"CAN rate\" objectType=\"7\" dataType=\"0005\" PDOmapping=\"no\" objFlags=\"00020000\" uniqueIDRef=\"UID_PARAM_240001\" />\n\t\t\t\t\t\t<CANopenSubObject subIndex=\"02\" name=\"RS232 rate\" objectType=\"7\" dataType=\"0005\" PDOmapping=\"no\" objFlags=\"00020001\" uniqueIDRef=\"UID_PARAM_240002\" />\n\t\t\t\t\t\t<CANopenSubObject subIndex=\"03\" name=\"Node ID\" objectType=\"7\" dataType=\"0005\" lowLimit=\"1\" highLimit=\"127\" accessType=\"rw\" defaultValue=\"1\" PDOmapping=\"no\" objFlags=\"00020001\" />\n\t\t\t\t\t\t<CANopenSubObject subIndex=\"04\" name=\"Communication settings\" objectType=\"7\" dataType=\"0007\" lowLimit=\"0\" highLimit=\"0x00078303\" accessType=\"rw\" defaultValue=\"0x00030302\" PDOmapping=\"no\" objFlags=\"00020000\" />\n\t\t\t\t\t\t<CANopenSubObject subIndex=\"05\" name=\"RS232 NetMode\" objectType=\"7\" dataType=\"0005\" lowLimit=\"0\" highLimit=\"255\" accessType=\"rw\" defaultValue=\"0\" PDOmapping=\"no\" objFlags=\"00020000\" />\n\t\t\t\t\t\t<CANopenSubObject subIndex=\"06\" name=\"ComState\" objectType=\"7\" dataType=\"0006\" accessType=\"ro\" PDOmapping=\"no\" objFlags=\"00020000\" />\n\t\t\t\t\t\t<CANopenSubObject subIndex=\"07\" name=\"ErrState\" objectType=\"7\" dataType=\"0006\" accessType=\"ro\" PDOmapping=\"no\" objFlags=\"0003\" />\n\t\t\t\t\t</CANopenObject>\n\t\t\t\t\t<CANopenObject index=\"2401\" name=\"USB Delay\" objectType=\"7\" dataType=\"0005\" lowLimit=\"0\" highLimit=\"255\" accessType=\"wo\" defaultValue=\"5\" PDOmapping=\"no\" objFlags=\"00020001\" />\n\t\t\t\t\t<CANopenObject index=\"2404\" name=\"FAID\" objectType=\"7\" dataType=\"0006\" lowLimit=\"0\" highLimit=\"65535\" accessType=\"wo\" defaultValue=\"0\" PDOmapping=\"no\" objFlags=\"00020003\" />\n\t\t\t\t\t<CANopenObject index=\"2405\" name=\"Bootloader SW version\" objectType=\"7\" dataType=\"0009\" accessType=\"ro\" defaultValue=\"0\" PDOmapping=\"no\" objFlags=\"00020000\" />\n\t\t\t\t\t<CANopenObject index=\"2406\" name=\"OD revision number\" objectType=\"7\" dataType=\"0007\" accessType=\"ro\" PDOmapping=\"no\" objFlags=\"00020000\" />\n\t\t\t\t\t<CANopenObject index=\"2407\" name=\"SW revision number\" objectType=\"7\" dataType=\"0007\" accessType=\"ro\" PDOmapping=\"no\" objFlags=\"00020000\" />\n\t\t\t\t\t<CANopenObject index=\"2408\" name=\"XDC Number\" objectType=\"7\" dataType=\"0007\" accessType=\"ro\" PDOmapping=\"no\" objFlags=\"00020000\" />\n\t\t\t\t\t<CANopenObject index=\"2410\" name=\"CAL access\" objectType=\"9\" subNumber=\"2\">\n\t\t\t\t\t\t<CANopenSubObject subIndex=\"00\" name=\"Number of entries\" objectType=\"7\" dataType=\"0005\" accessType=\"ro\" defaultValue=\"1\" PDOmapping=\"no\" />\n\t\t\t\t\t\t<CANopenSubObject subIndex=\"01\" name=\"CAL key\" objectType=\"7\" dataType=\"0007\" lowLimit=\"0\" highLimit=\"4294967295\" accessType=\"rw\" PDOmapping=\"no\" objFlags=\"00020000\" />\n\t\t\t\t\t</CANopenObject>\n\t\t\t\t\t<CANopenObject index=\"2500\" name=\"ADC scaling (offset|gain)\" objectType=\"9\" subNumber=\"15\">\n\t\t\t\t\t\t<CANopenSubObject subIndex=\"00\" name=\"Number of entries\" objectType=\"7\" dataType=\"0005\" accessType=\"ro\" defaultValue=\"14\" PDOmapping=\"no\" />\n\t\t\t\t\t\t<CANopenSubObject subIndex=\"01\" name=\"IA scaling\" objectType=\"7\" dataType=\"0007\" lowLimit=\"0x0\" accessType=\"ro\" PDOmapping=\"no\" objFlags=\"00020000\" />\n\t\t\t\t\t\t<CANopenSubObject subIndex=\"02\" name=\"IB scaling\" objectType=\"7\" dataType=\"0007\" lowLimit=\"0x0\" accessType=\"ro\" PDOmapping=\"no\" objFlags=\"00020000\" />\n\t\t\t\t\t\t<CANopenSubObject subIndex=\"03\" name=\"IC scaling\" objectType=\"7\" dataType=\"0007\" lowLimit=\"0x0\" accessType=\"ro\" PDOmapping=\"no\" objFlags=\"00020000\" />\n\t\t\t\t\t\t<CANopenSubObject subIndex=\"04\" name=\"Hall A scaling\" objectType=\"7\" dataType=\"0007\" lowLimit=\"0x0\" accessType=\"ro\" PDOmapping=\"no\" objFlags=\"00020000\" />\n\t\t\t\t\t\t<CANopenSubObject subIndex=\"05\" name=\"Hall B scaling\" objectType=\"7\" dataType=\"0007\" lowLimit=\"0x0\" accessType=\"ro\" PDOmapping=\"no\" objFlags=\"00020000\" />\n\t\t\t\t\t\t<CANopenSubObject subIndex=\"06\" name=\"Hall C scaling\" objectType=\"7\" dataType=\"0007\" lowLimit=\"0x0\" accessType=\"ro\" PDOmapping=\"no\" objFlags=\"00020000\" />\n\t\t\t\t\t\t<CANopenSubObject subIndex=\"07\" name=\"Analog input 1 scaling\" objectType=\"7\" dataType=\"0007\" lowLimit=\"0x0\" accessType=\"ro\" PDOmapping=\"no\" objFlags=\"00020000\" />\n\t\t\t\t\t\t<CANopenSubObject subIndex=\"08\" name=\"Analog input 2 scaling\" objectType=\"7\" dataType=\"0007\" lowLimit=\"0x0\" accessType=\"ro\" PDOmapping=\"no\" objFlags=\"00020000\" />\n\t\t\t\t\t\t<CANopenSubObject subIndex=\"09\" name=\"Uel scaling\" objectType=\"7\" dataType=\"0007\" lowLimit=\"0x0\" accessType=\"ro\" PDOmapping=\"no\" objFlags=\"00020000\" />\n\t\t\t\t\t\t<CANopenSubObject subIndex=\"0A\" name=\"Udc scaling\" objectType=\"7\" dataType=\"0007\" lowLimit=\"0x0\" accessType=\"ro\" PDOmapping=\"no\" objFlags=\"00020000\" />\n\t\t\t\t\t\t<CANopenSubObject subIndex=\"0B\" name=\"Internal temperature scaling\" objectType=\"7\" dataType=\"0007\" lowLimit=\"0x0\" accessType=\"ro\" PDOmapping=\"no\" objFlags=\"00020000\" />\n\t\t\t\t\t\t<CANopenSubObject subIndex=\"0C\" name=\"External temperature scaling\" objectType=\"7\" dataType=\"0007\" lowLimit=\"0x0\" accessType=\"ro\" PDOmapping=\"no\" objFlags=\"00020000\" />\n\t\t\t\t\t\t<CANopenSubObject subIndex=\"0D\" name=\"Motor NTC gain\" objectType=\"7\" dataType=\"0004\" lowLimit=\"0x80000000\" accessType=\"ro\" PDOmapping=\"no\" objFlags=\"00030000\" />\n\t\t\t\t\t
